vi "Power Serial.vi"(7 "VISA Resource Address":i32=5, 8 "error in (no error)":errorcluster, 9 "Rd?":bool, 10 "Delay":u32=200, 11 "IN":string) -> (0 "error out":errorcluster, 3 "OUT":string)   [LabVIEW 2009]
doc: "程控电源控制命令子程序\n功能描述：通过串口的读写完成对电源的命令的发送。\n输入：命令，延时，读写控制，串口号，错误信息\n输出：命令，错误信息"
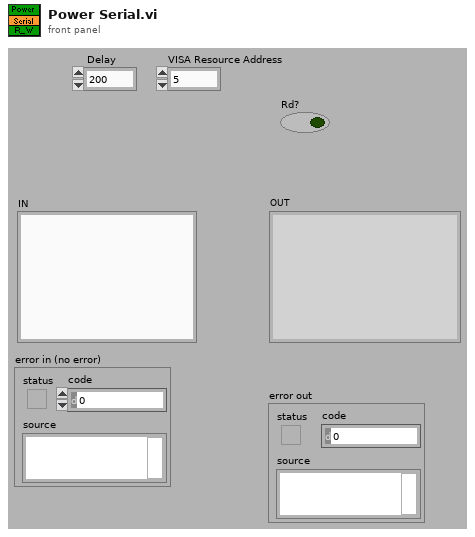
[diagram p1: front panel]
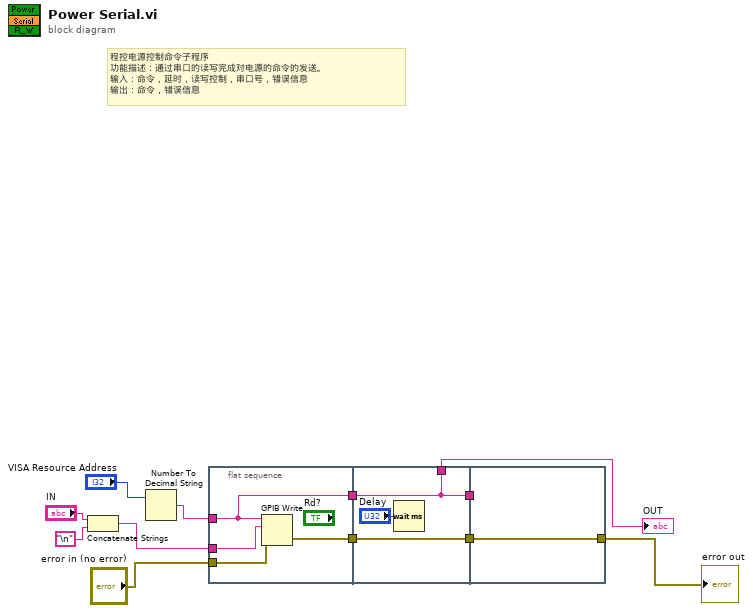
[diagram p0: block diagram]
diagram:
  # "程控电源控制命令子程序\n功能描述：通过串口的读写完成对电源的命令的发送。\n输入：命令，延时，读写控制，串口号，错误信息\n输出：命令，错误信息"
  n1 = Concatenate Strings("IN", "\n") -> (w5:string)
  n2 = Number To Decimal String(number="VISA Resource Address") -> (decimal integer string=w7:string)  [unwired: 1 out]
  n3 = flat-sequence {
    tunnel: w7 -> [w15]
    tunnel: w5 -> [w16]
    tunnel: [w15] -> w12
    tunnel: "error in (no error)" -> [w14]
    tunnel: [w13] -> w11
    tunnel: [w17] -> w10
    tunnel: w12 -> [w17]
    tunnel: [w19] -> w9
    tunnel: w11 -> [w19]
    tunnel: [w17] -> w2
    tunnel: w10 -> [_]
    tunnel: w9 -> [w20]
    tunnel: [w20] -> w1
    frame #0 {
      n4 = GPIB Write(0:w15, 1:w16, 3:w14) -> (6:w13:errorcluster)  [unwired: 3 out]
    }
    frame #1 {
      n5 = Wait (ms)(milliseconds to wait="Delay") -> ()  [unwired: 1 out]
    }
    frame #2 {
    }
  }
  "OUT" <- w2
  "error out" <- w1
